vi "Periodic Tasks.vi"(8 "error in":errorcluster) -> ()   [LabVIEW 2020]
doc: "This VI runs in parallel to other tasks. It can contain as many user-defined periodic loops as you need. These can carry out PID or other sorts of timed response."
uses:
  <vilib>/Rock Robotics/WPI/Utilities/WPI_GetSetVariantRefNum.vi
  MyGlobal.vi
panel:
  out "winch 2":dbl
  out "winch":dbl
  out "Deploiement ramasse balle":dbl
  out "ramasse balle":dbl
  out "force feed balle":dbl
  out "force moteurs lance balle":dbl
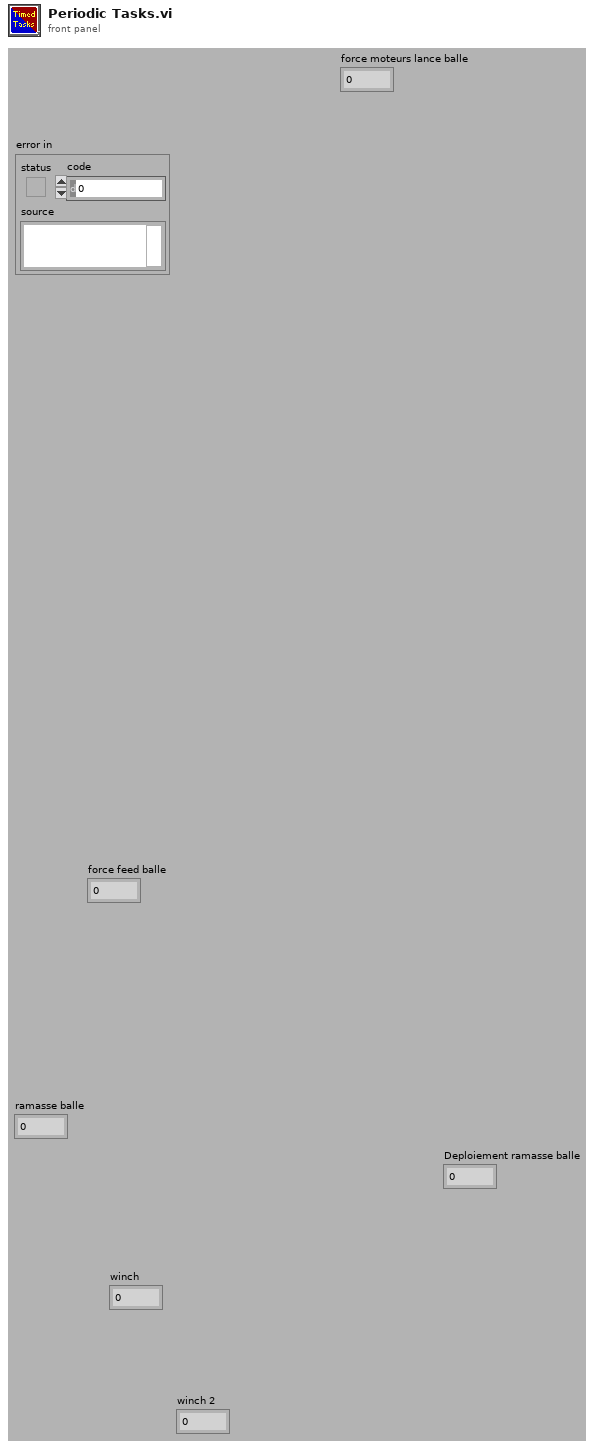
[diagram p1: front panel]
types:
  T1 = typedef "WPI_JoystickDevRef.ctl" = cluster{"Device":T2}
  T2 = typedef "WPI_JoystickDeviceEnum.ctl" = enum16{"USB 0", "USB 1", "USB 2", "USB 3", "USB 4", "USB 5"}
  T3 = typedef "WPI_RobotDriveDevRef.ctl" = cluster{"DevStatus":errorcluster, "Motors[]":T4[], "Square Inputs":bool, "Max Output":dbl}
  T4 = typedef "WPI_MotorControlDeviceRef.ctl" = cluster{"DeviceStatus":errorcluster, "Type":T5, "PWM":cluster{"PWM Channel":T6, "DeadBand":T7}, "CAN":cluster{"Device Number":u8, "SetOutput VI Ref":variant, "GetOutput VI Ref":variant, "Enable VI Ref":variant, "Disable VI Ref":variant, "Data":variant}, "Invert":bool, "DIO PWM":cluster{"PWM \"Enable\" Channel":T6, "DIOChannel":T8, "PWM Rate":dbl}}
  T5 = typedef "WPI_MotorControlType.ctl" = enum16{"PWM", "CAN", "DIO PWM"}
  T6 = typedef "FPGA_DIOPWMChannel.ctl" = enum8{"PWM 0", "PWM 1", "PWM 2", "PWM 3", "PWM 4", "PWM 5", "PWM 6", "PWM 7", "PWM 8", "PWM 9", "PWM MXP 0", "PWM MXP 1", "PWM MXP 2", "PWM MXP 3", "PWM MXP 4", "PWM MXP 5", "PWM MXP 6", "PWM MXP 7", "PWM MXP 8", "PWM MXP 9", "Invalid"}
  T7 = typedef "WPI_PWMDeadband.ctl" = cluster{"Name":string, "maxPositivePwm":i32, "minPositivePwm":i32, "centerPwm":i32, "maxNegativePwm":i32, "minNegativePwm":i32, "angularRange":u16}
  T8 = typedef "FPGA_DIOChannel.ctl" = enum8{"DIO 0", "DIO 1", "DIO 2", "DIO 3", "DIO 4", "DIO 5", "DIO 6", "DIO 7", "DIO 8", "DIO 9", "DIO MXP 0", "DIO MXP 1", "DIO MXP 2", "DIO MXP 3", "DIO MXP 4", "DIO MXP 5", "DIO MXP 6", "DIO MXP 7", "DIO MXP 8", "DIO MXP 9", "DIO MXP 10", "DIO MXP 11", "DIO MXP 12", "DIO MXP 13", "DIO MXP 14", "DIO MXP 15", "SPI Port CS1", "SPI Port CS2", "SPI Port CS3", "SPI Port MISO", "SPI Port MOSI", "Invalid"}
  T9 = cluster{"JoystickDevRef":T1, "RobotDriveDevRef":T3}
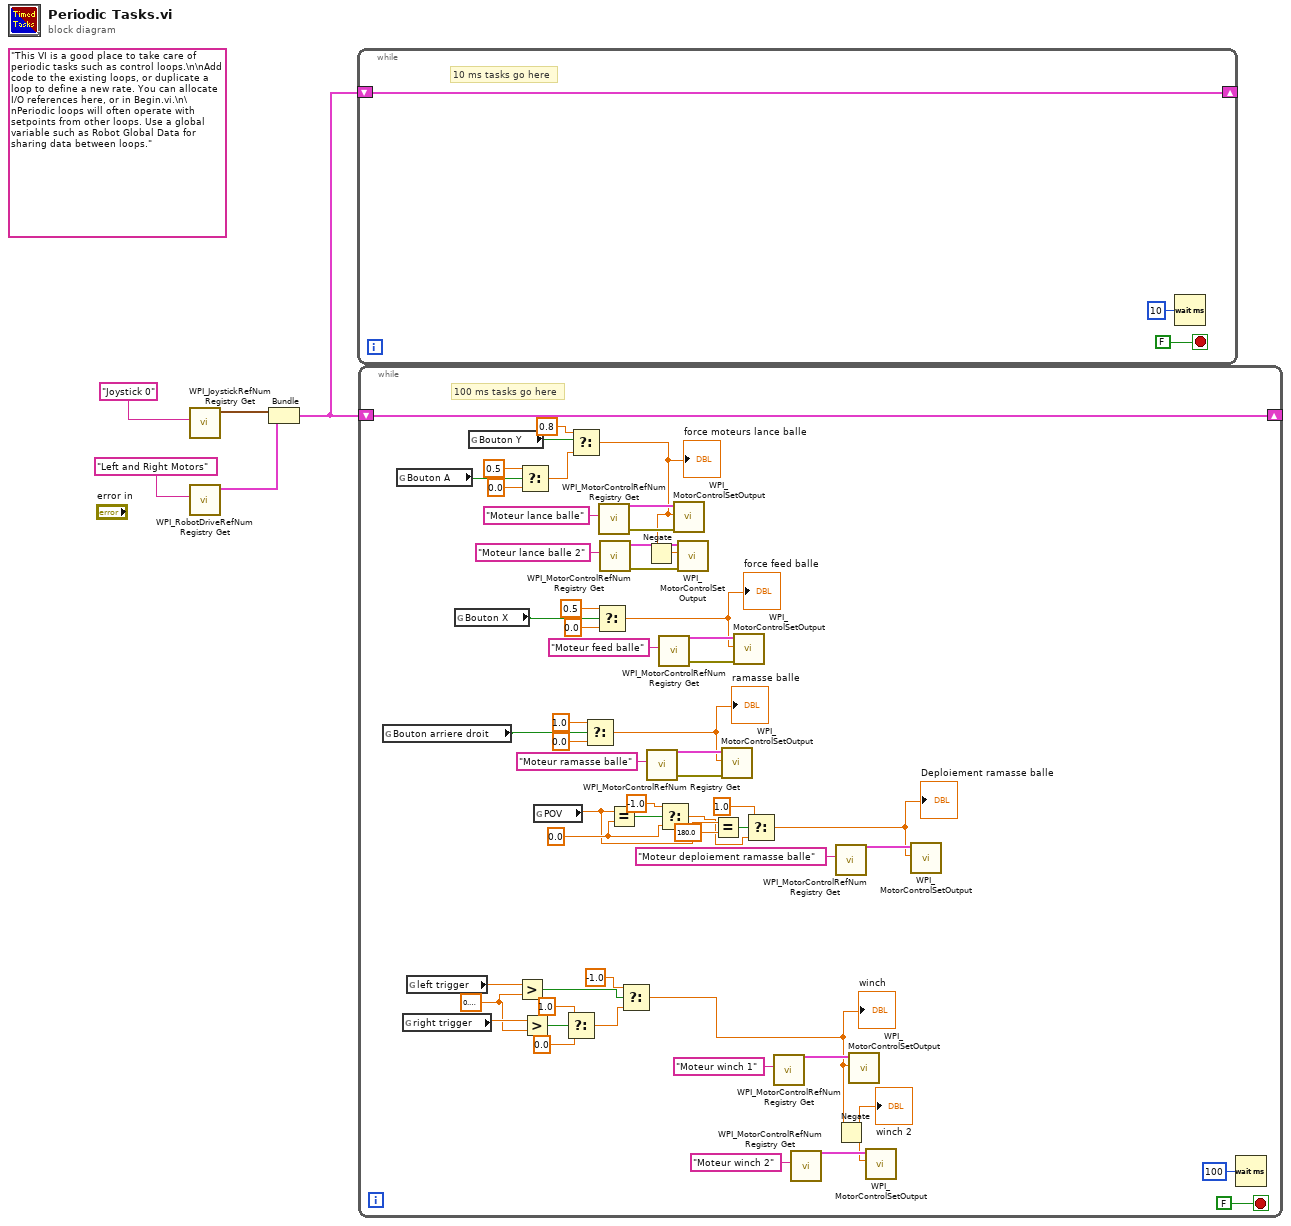
[diagram p0: block diagram]
diagram:
  (unwired) "This VI is a good place to take care of periodic tasks such as control loops.\n\nAdd code to the existing loops, or duplicate a loop to define a new rate. You can allocate I/O references here, or in Begin.vi.\n\nPeriodic loops will often operate with setpoints from other loops. Use a global variable such as Robot Global Data for sharing data between loops."
  n1 = call <vilib>:"WPI_JoystickRefNum Registry Get.vi"("refnum name"="Joystick 0") -> ("JoystickDevRef"=w3:T1)  [unwired: 1 in, 9 out]
  n2 = call <vilib>:"WPI_RobotDriveRefNum Registry Get.vi"("refnum name"="Left and Right Motors") -> ("RobotDriveDevRef"=w2:T3)  [unwired: 1 in, 9 out]
  n3 = Bundle("JoystickDevRef"=w3, "RobotDriveDevRef"=w2) -> (w1:T9)  [unwired: 1 out]
  n4 = while {
    shift-right: [w6] -> _
    shift-left: w1 -> [w6]
    stop <- FALSE stop-if-true
    # "10 ms tasks go here"
    n5 = Wait (ms)(milliseconds to wait=u32 10) -> ()  [unwired: 1 out]
  }
  n6 = while {
    shift-right: [w63] -> _
    shift-left: w1 -> [w63]
    stop <- FALSE stop-if-true
    w21 = sgl 0.2 ("y")
    w32 = 0.0
    # "100 ms tasks go here"
    n7 = global read "MyGlobal.vi" "Bouton arriere droit"() -> (w35:bool)
    n8 = global read "MyGlobal.vi" "Bouton A"() -> (w62:bool)
    n9 = global read "MyGlobal.vi" "right trigger"() -> (w22:sgl)
    n10 = global read "MyGlobal.vi" "left trigger"() -> (w23:sgl)
    n11 = global read "MyGlobal.vi" "Bouton X"() -> (w46:bool)
    n12 = global read "MyGlobal.vi" "Bouton Y"() -> (w58:bool)
    n13 = Greater?(x=w23, y=w21) -> (0:w18:bool)
    n14 = Select(t=0.5, s=w62, f=0.0) -> (s? t:f=w57:dbl)
    n15 = Greater?(x=w22, y=w21) -> (0:w20:bool)
    n16 = global read "MyGlobal.vi" "POV"() -> (w30:sgl)
    n17 = Select(t=1.0, s=w20, f=0.0) -> (s? t:f=w19:dbl)
    n18 = Select(t=0.8, s=w58, f=w57) -> (s? t:f=w50:dbl)
    "force moteurs lance balle" <- w50
    n19 = Select(t=1.0, s=w35, f=0.0) -> (s? t:f=w36:dbl)
    "ramasse balle" <- w36
    n20 = Select(t=0.5, s=w46, f=0.0) -> (s? t:f=w42:dbl)
    "force feed balle" <- w42
    n21 = call <vilib>:"WPI_MotorControlRefNum Registry Get.vi"("refnum name"="Moteur lance balle") -> ("error out"=w53:errorcluster, "MotorControlDevRef"=w54:T4)  [unwired: 9 in]
    n22 = call <vilib>:"WPI_MotorControlRefNum Registry Get.vi"("refnum name"="Moteur lance balle 2") -> ("error out"=w51:errorcluster, "MotorControlDevRef"=w52:T4)  [unwired: 9 in]
    n23 = Equal?(x=w30, y=w32) -> (x = y?=w34:bool)
    n24 = Select(t=-1.0, s=w18, f=w19) -> (s? t:f=w10:dbl)
    "winch" <- w10
    n25 = Negate(x=w50) -> (-x=w49:dbl)
    n26 = call <vilib>:"WPI_MotorControlRefNum Registry Get.vi"("refnum name"="Moteur ramasse balle") -> ("error out"=w37:errorcluster, "MotorControlDevRef"=w38:T4)  [unwired: 9 in]
    n27 = call <vilib>:"WPI_MotorControlRefNum Registry Get.vi"("refnum name"="Moteur feed balle") -> ("error out"=w43:errorcluster, "MotorControlDevRef"=w44:T4)  [unwired: 9 in]
    n28 = Select(t=-1.0, s=w34, f=w32) -> (s? t:f=w27:dbl)
    n29 = call <vilib>:"WPI_MotorControlSetOutput.vi"("error in (no error)"=w53, "Output"=w50, "MotorControlDevRef"=w54) -> ()  [unwired: 6 in, 3 out]
    n30 = call <vilib>:"WPI_MotorControlSetOutput.vi"("error in (no error)"=w51, "Output"=w49, "MotorControlDevRef"=w52) -> ()  [unwired: 6 in, 3 out]
    n31 = Equal?(x=w30, y=sgl 180.0) -> (x = y?=w31:bool)
    n32 = call <vilib>:"WPI_MotorControlSetOutput.vi"("error in (no error)"=w37, "Output"=w36, "MotorControlDevRef"=w38) -> ()  [unwired: 6 in, 3 out]
    n33 = call <vilib>:"WPI_MotorControlSetOutput.vi"("error in (no error)"=w43, "Output"=w42, "MotorControlDevRef"=w44) -> ()  [unwired: 6 in, 3 out]
    n34 = Select(t=1.0, s=w31, f=w27) -> (s? t:f=w24:dbl)
    "Deploiement ramasse balle" <- w24
    n35 = call <vilib>:"WPI_MotorControlRefNum Registry Get.vi"("refnum name"="Moteur winch 1") -> ("MotorControlDevRef"=w13:T4)  [unwired: 9 in, 1 out]
    n36 = call <vilib>:"WPI_MotorControlRefNum Registry Get.vi"("refnum name"="Moteur winch 2") -> ("MotorControlDevRef"=w11:T4)  [unwired: 9 in, 1 out]
    n37 = call <vilib>:"WPI_MotorControlRefNum Registry Get.vi"("refnum name"="Moteur deploiement ramasse balle") -> ("MotorControlDevRef"=w25:T4)  [unwired: 9 in, 1 out]
    n38 = Negate(x=w10) -> (-x=w9:dbl)
    "winch 2" <- w9
    n39 = call <vilib>:"WPI_MotorControlSetOutput.vi"("Output"=w10, "MotorControlDevRef"=w13) -> ()  [unwired: 7 in, 3 out]
    n40 = call <vilib>:"WPI_MotorControlSetOutput.vi"("Output"=w9, "MotorControlDevRef"=w11) -> ()  [unwired: 7 in, 3 out]
    n41 = call <vilib>:"WPI_MotorControlSetOutput.vi"("Output"=w24, "MotorControlDevRef"=w25) -> ()  [unwired: 7 in, 3 out]
    n42 = Wait (ms)(milliseconds to wait=u32 100) -> ()  [unwired: 1 out]
  }
